vi "ExSubSetTemp.vi"(2 "error in (no error)":errorcluster, 3 "Temperature":dbl format="%.2f", 4 "CameraHandle":u32) -> (0 "error out":errorcluster, 1 "Camera Handle":u32)   [LabVIEW 2010]
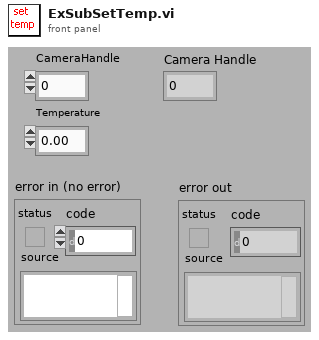
[diagram p1: front panel]
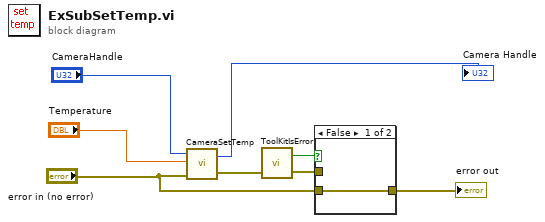
[diagram p0: block diagram]
diagram:
  n1 = call <userlib>:"CameraSetTemp.vi"("error in (no error)"="error in (no error)", "Temperature"="Temperature", "Camera Handle"="CameraHandle") -> ("error out"=w6:errorcluster, "Camera Handle"=→"Camera Handle":u32)
  n2 = call <userlib>:"ToolKitIsError.vi"("error in"=w6) -> ("error out"=w7:errorcluster, "Error Flag"=w8:bool)  [unwired: 1 in]
  n3 = case shown="False" w8 {
    tunnel: w7 -> [_ w10]
    tunnel: [w9 w10] -> w1
    tunnel: "error in (no error)" -> [w9 _]
    frame False {
    }
    frame True {
    }
  }
  "error out" <- w1
